vi "OnOff Write.vi"(8 "error in":errorcluster, 10 "OnOff STS":i32, 11 "OnOff in":refnum<class "OnOff.lvclass">) -> (0 "error out":errorcluster, 3 "OnOff out":refnum<class "OnOff.lvclass">)   [LabVIEW 2023, in "OnOff.lvclass"]
uses:
  OnOff.lvclass
  OnOff.lvclass/OnOff.ctl
  <vilib>/ADAS Replay HIL/Channels/Tag Wrapper/Polymorphic/Write Channel (I32).vi
  <vilib>/ADAS Replay HIL/Channels/Tag Wrapper/Polymorphic/Write Channel (I32).vi/cccb8e89-591f-4bb4-9d4e-ae06ba1f5498.vi
  <vilib>/ADAS Replay HIL/Channels/Tag Wrapper/Polymorphic/Write Channel (I32).vi/cccb8e89-591f-4bb4-9d4e-ae06ba1f5498.vi/4bc1c15b-36ab-481f-b8dd-c64075ce723a.vi
  <vilib>/ADAS Replay HIL/Channels/Tag Wrapper/Polymorphic/Write Channel (I32).vi/cccb8e89-591f-4bb4-9d4e-ae06ba1f5498.vi/d83cb72b-7713-41fc-a3d1-682de79cf574.vi
  <vilib>/ADAS Replay HIL/Channels/Tag Wrapper/Tag Wrapper.lvlib
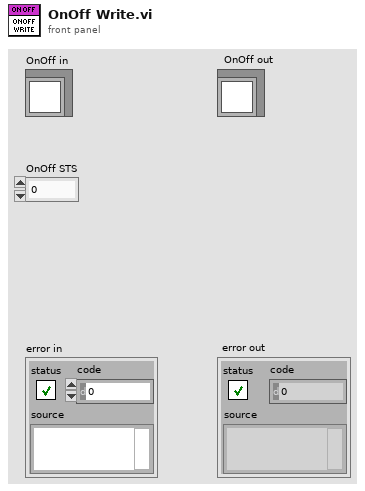
[diagram p1: front panel]
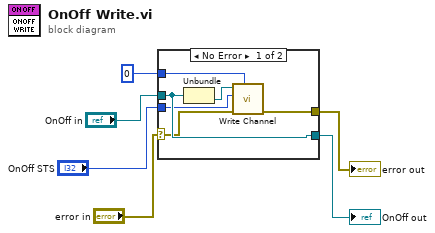
[diagram p0: block diagram]
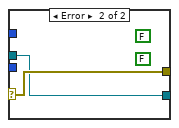
[diagram p2: hidden frame]
diagram:
  n1 = case shown="No Error" "error in" {
    selector: "error in" -> [w10 w14]
    tunnel: [w9 w14] -> w5
    tunnel: "OnOff in" -> [w12 w13]
    tunnel: [w12 w13] -> w3
    tunnel: "OnOff STS" -> [w8 _]
    tunnel: 0 ("Timeout (ms)") -> [w7 _]
    frame No Error {
      n2 = Unbundle(w12) -> (w11:refnum<k21>)  [unwired: 1 out]
      n3 = call-poly <vilib>:"Write Channel.vi"("Timeout (ms)"=w7, "error in"=w10, "Value to Write"=w8, "ADAS HIL Channel in"=w11) -> ("error out"=w9:errorcluster)  [unwired: 5 in, 2 out]
    }
    frame Error {
      (unwired) FALSE
      (unwired) FALSE ("changed or first call?")
    }
  }
  "error out" <- w5
  "OnOff out" <- w3
